vi "ReadWrite.EngineData.vi"(8 "error in":errorcluster, 10 "Force":bool, 11 "ReadWrite in":refnum<class "ReadWrite.lvclass">) -> (0 "error out":errorcluster, 3 "ReadWrite out":refnum<class "ReadWrite.lvclass">)   [LabVIEW 2027, in "Data Access Engine.lvlib" / "ReadWrite.lvclass"]
uses:
  ReadWrite.lvclass
  ReadWrite.lvclass/ReadWrite.ctl
  <vilib>/NI VeriStand/Custom Device API/Global Data Refs.vi
  <vilib>/NI VeriStand/Custom Device API/Custom Device API.lvlib
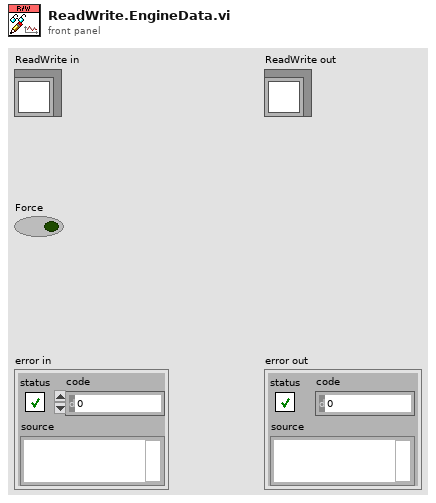
[diagram p1: front panel]
types:
  T1 = typedef "Custom Device API.lvlib/Data Reference.ctl" = i32
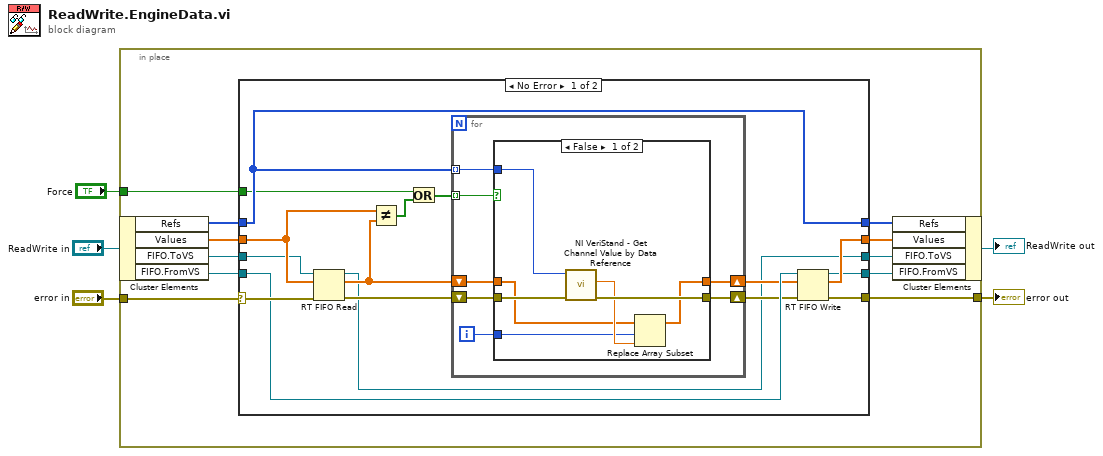
[diagram p0: block diagram]
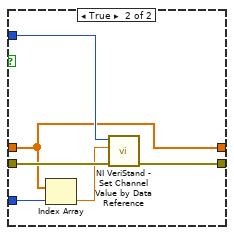
[diagram p2: hidden frame]
diagram:
  n1 = in-place {
    in-place-border: [w16] -> w5
    in-place-border: "error in" -> [w11]
    in-place-border: "Force" -> [w6]
    n2 = in-place-cluster #1("ReadWrite in") -> ("Refs"=w15:T1[], "Values"=w14:dbl[], "FIFO.ToVS"=w9:refnum<k33>, "FIFO.FromVS"=w10:refnum<k33>)
    n3 = case shown="No Error" w11 {
      selector: w11 -> [w29 w56]
      tunnel: [w31 w56] -> w16
      tunnel: [w23 w55] -> w13
      tunnel: w15 -> [w22 w54]
      tunnel: w14 -> [w28 w55]
      tunnel: [w22 w54] -> w12
      tunnel: w9 -> [w26 w53]
      tunnel: w10 -> [w25 w52]
      tunnel: [w20 w53] -> w8
      tunnel: [w21 w52] -> w7
      tunnel: w6 -> [w19 _]
      frame No Error {
        n4 = RT FIFO Read(0:w26, 1:w28, 3:w29) -> (8:w20:refnum<k33>, 9:w27:dbl[], 11:w30:errorcluster)  [unwired: 1 in, 2 out]
        n5 = Not Equal?(x=w28, y=w27) -> (x != y?=w18:bool[])
        n6 = Or(x=w19, y=w18) -> (x .or. y?=w17:bool[])
        n7 = for {
          shift-right: [w38] -> w24
          shift-left: w30 -> [w37]
          tunnel: w17 -> [w34] mode=indexing
          tunnel: w22 -> [w35] mode=indexing
          shift-right: [w32] -> w23
          shift-left: w27 -> [w36]
          i -> [w33]
          n8 = case shown="False" w34 {
            tunnel: w36 -> [w40 w46]
            tunnel: [w43 w50] -> w38
            tunnel: w37 -> [w44 w51]
            tunnel: w35 -> [w45 w49]
            tunnel: w33 -> [w41 w48]
            tunnel: [w39 w46] -> w32
            frame False {
              n9 = call <vilib>:"NI VeriStand - Get Channel Value by Data Reference.vi"("error in (no error)"=w44, "Data Reference in"=w45) -> ("error out"=w43:errorcluster, "Value"=w42:dbl)  [unwired: 8 in]
              n10 = Replace Array Subset(array=w40, new element=w42, index=w41) -> (w39:dbl[])
            }
            frame True {
              n11 = Index Array(array=w46, index=w48) -> (element=w47:dbl)
              n12 = call <vilib>:"NI VeriStand - Set Channel Value by Data Reference.vi"("error in (no error)"=w51, "Value"=w47, "Data Reference in"=w49) -> ("error out"=w50:errorcluster)  [unwired: 8 in]
            }
          }
        }
        n13 = RT FIFO Write(0:w25, 1:w23, 3:w24) -> (8:w21:refnum<k33>, 11:w31:errorcluster)  [unwired: 2 in, 2 out]
      }
      frame Error {
      }
    }
    n14 = in-place-cluster #1("Refs"=w12, "Values"=w13, "FIFO.ToVS"=w8, "FIFO.FromVS"=w7) -> (→"ReadWrite out":refnum<class "ReadWrite.lvclass">)
  }
  "error out" <- w5
